vi "Set Panel Info.vi"(6 "VI Refnum":refnum<vi>, 7 "Parent Panel":string, 8 "error in (no error)":errorcluster, 10 "Panel Updater":refnum<class "Panel Updater.lvclass">, 11 "Panel Helper in":refnum<class "Panel Helper.lvclass">) -> (0 "error out":errorcluster)   [LabVIEW 2020, in "Panel.lvlib" / "Panel Helper.lvclass"]
doc: "Sets the VI ref. Automatically initializes the Panel Helper if needed.\n----\nCopyright: MGI 2016\nAuthor: Derek Trepanier"
uses:
  <vilib>/MGI/Panel Manager/Panel/Panel Helper/Panel Helper.lvclass
  <vilib>/MGI/Panel Manager/Panel/Panel Updater/Panel Updater.lvclass
  <vilib>/MGI/Panel Manager/Panel/Panel Helper/Events.ctl
  <vilib>/MGI/Panel Manager/Panel/Panel Helper/Panel Helper.lvclass/Panel Helper.ctl
  <vilib>/MGI/Panel Manager/Panel/Deferer/Deferer.lvclass
  <vilib>/MGI/Panel Manager/Panel/Panel Registry/Panel Registry.lvclass
  <vilib>/MGI/Panel Manager/Panel/Panel.lvlib
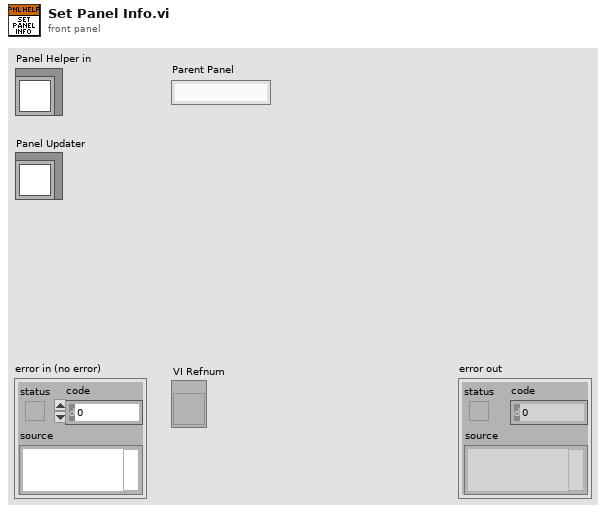
[diagram p1: front panel]
types:
  T1 = typedef "Panel.lvlib/Panel Helper.lvclass/Events.ctl" = enum16{"Initialized", "Shown", "Hidden", "Closed"}
  T2 = typedef "Panel.lvlib/Panel Helper.lvclass/Panel Events.ctl" = cluster{"My Panel":refnum<user-event>, "Top Level Initialized":refnum<user-event>}
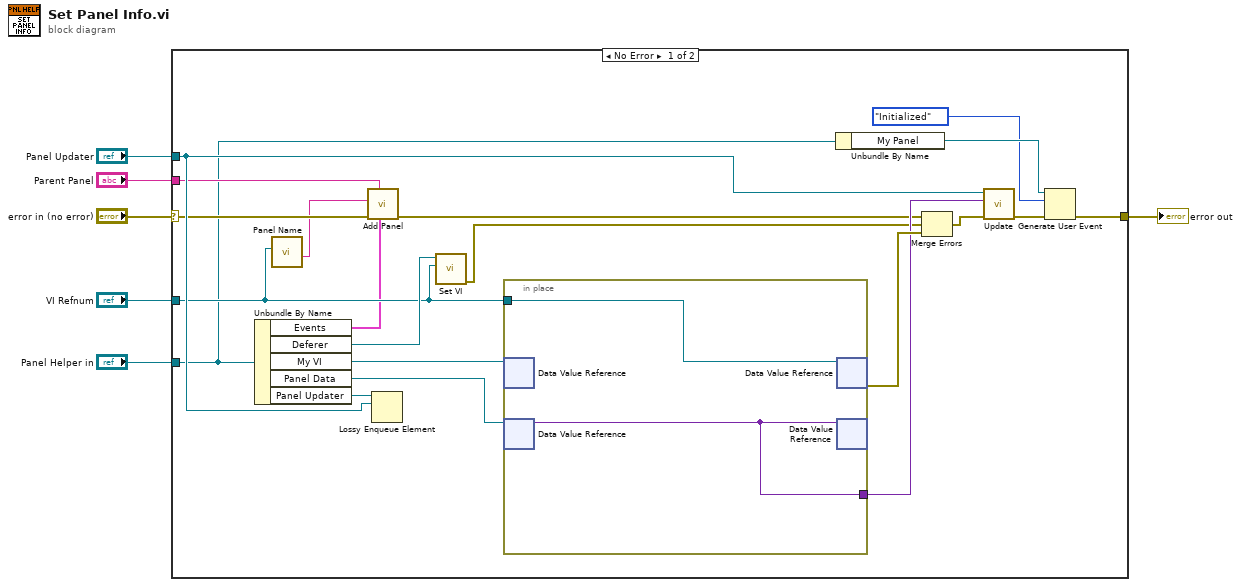
[diagram p0: block diagram]
diagram:
  n1 = case shown="No Error" "error in (no error)" {
    selector: "error in (no error)" -> [w17 w29]
    tunnel: [w10 w29] -> w5
    tunnel: "Panel Helper in" -> [w12 _]
    tunnel: "VI Refnum" -> [w15 _]
    tunnel: "Panel Updater" -> [w20 _]
    tunnel: "Parent Panel" -> [w14 _]
    frame No Error {
      n2 = Unbundle By Name(w12) -> ("Events"=w13:T2, "Deferer"=w19:refnum<class "Deferer.lvclass">, "My VI"=w26:refnum<data-value>, "Panel Data"=w24:refnum<data-value>, "Panel Updater"=w23:refnum<queue>)
      n3 = call <vilib>:"Panel Name.vi"("VI in"=w15) -> ("Name"=w7:string)  [unwired: 9 in, 1 out]
      n4 = call <vilib>:"Add Panel.vi"("Events"=w13, "Parent"=w14, "error in (no error)"=w17, "Panel"=w7) -> ("error out"=w16:errorcluster)  [unwired: 7 in]
      n5 = Lossy Enqueue Element(queue=w23, element=w20) -> ()  [unwired: 1 in, 4 out]
      n6 = call <vilib>:"Set VI.vi"("VI ref"=w15, "Deferer in"=w19) -> ("error out"=w18:errorcluster)  [unwired: 9 in]
      n7 = in-place {
        in-place-border: w15 -> [w28]
        in-place-border: [w27] -> w22
        n8 = in-place-dvr #1(w26) -> ()  [unwired: 2 out]
        n9 = in-place-dvr #2(w24) -> (w27:variant)  [unwired: 1 out]
        n10 = in-place-dvr #1(w28) -> (w25:errorcluster)  [unwired: 1 out]
        n11 = in-place-dvr #2(w27) -> ()  [unwired: 2 out]
      }
      n12 = Unbundle By Name(w12) -> ("My Panel"=w9:refnum<user-event>)
      n13 = Merge Errors(w16, w18, w25) -> (w21:errorcluster)
      n14 = call-dynamic "Update.vi"("error in (no error)"=w21, "Panel Data"=w22, "Panel Updater in"=w20) -> ("error out"=w11:errorcluster)  [unwired: 8 in]
      n15 = Generate User Event(user event=w9, event data cluster=Events."Initialized" ("event data"), error in=w11) -> (error out=w10:errorcluster)  [unwired: 1 in, 1 out]
    }
    frame Error {
    }
  }
  "error out" <- w5
